vi "do all three.vi"(6 "Gyro Target":dbl, 7 "Max Time":dbl, 8 "X Target":dbl, 9 "Y Target":dbl, 10 "Encoders In":T1, 11 "PID Gains In":T2={"X PID"={"proportional gain (Kc)"=0.02000000000000001, "integral time (Ti, min)"=0.0, "derivative time (Td, min)"=0.0}, "Y PID"={"proportional gain (Kc)"=0.02000000000000001, "integral time (Ti, min)"=0.0, "derivative time (Td, min)"=0.0}, "Z PID"={"proportional gain (Kc)"=0.02000000000000001, "integral time (Ti, min)"=0.0, "derivative time (Td, min)"=0.0}} {"Z PID"."derivative time (Td, min)" format="%.3f"; "Z PID"."integral time (Ti, min)" format="%.3f"; "Z PID"."proportional gain (Kc)" format="%.3f"; "Y PID"."derivative time (Td, min)" format="%.3f"; "Y PID"."integral time (Ti, min)" format="%.3f"; "Y PID"."proportional gain (Kc)" format="%.3f"; "X PID"."derivative time (Td, min)" format="%.3f"; "X PID"."integral time (Ti, min)" format="%.3f"; "X PID"."proportional gain (Kc)" format="%.3f"}) -> (2 "Encoders Out":T1, 3 "PID Gains Out":T2={"X PID"={"proportional gain (Kc)"=0.02000000000000001, "integral time (Ti, min)"=0.0, "derivative time (Td, min)"=0.0}, "Y PID"={"proportional gain (Kc)"=0.02000000000000001, "integral time (Ti, min)"=0.0, "derivative time (Td, min)"=0.0}, "Z PID"={"proportional gain (Kc)"=0.02000000000000001, "integral time (Ti, min)"=0.0, "derivative time (Td, min)"=0.0}} {"Z PID"."derivative time (Td, min)" format="%.3f"; "Z PID"."integral time (Ti, min)" format="%.3f"; "Z PID"."proportional gain (Kc)" format="%.3f"; "Y PID"."derivative time (Td, min)" format="%.3f"; "Y PID"."integral time (Ti, min)" format="%.3f"; "Y PID"."proportional gain (Kc)" format="%.3f"; "X PID"."derivative time (Td, min)" format="%.3f"; "X PID"."integral time (Ti, min)" format="%.3f"; "X PID"."proportional gain (Kc)" format="%.3f"})   [LabVIEW 2018]
uses:
  <vilib>/addons/control/pid/NI_PID_pid.lvlib
  <vilib>/addons/control/pid/pid.llb/PID (DBL).vi
  Robot Global Data.vi
  SubSystems/Robot Information/Robot Information Global.vi
panel:
  in  "rest time":u32
  in  "Movement":enum16{"0", "1", "2", "3", "4", "5"}(ring)
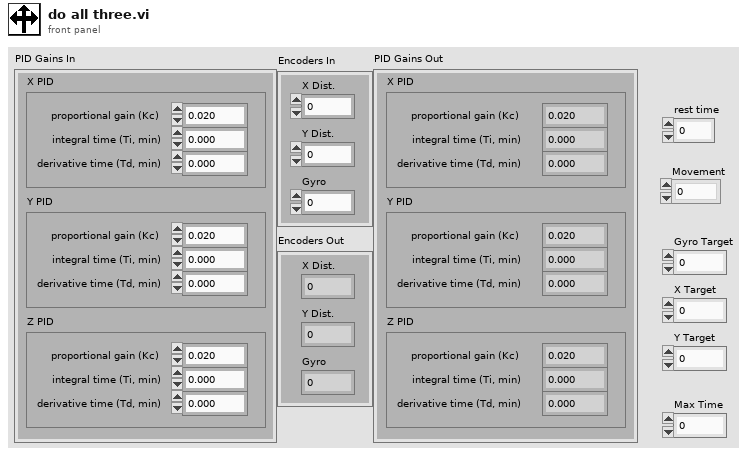
[diagram p1: front panel]
types:
  T1 = cluster{"X Dist.":dbl, "Y Dist.":dbl, "Gyro":dbl}
  T2 = cluster{"X PID":cluster{"proportional gain (Kc)":dbl, "integral time (Ti, min)":dbl, "derivative time (Td, min)":dbl}, "Y PID":cluster{"proportional gain (Kc)":dbl, "integral time (Ti, min)":dbl, "derivative time (Td, min)":dbl}, "Z PID":cluster{"proportional gain (Kc)":dbl, "integral time (Ti, min)":dbl, "derivative time (Td, min)":dbl}}
  T3 = enum16{"HP, Far-Top rocket, Lvl2 Right", "HP, Far-Top rocket, Lvl2 Left", "HP, Far-Top rocket, Lvl1 Right", "HP, Far-Top rocket, Lvl1 Left", "HP, Both-Top rocket, Lvl2 Right", "HP, Both-Top rocket, Lvl2 Left", "HP, Both-Top rocket, Lvl1 Right", "HP, Both-Top rocket, Lvl1 Left", "HP, Near cargo, Lvl2 ", "HP, Near cargo, Lvl1", "HP, Far cargo, Lvl2 ", "HP, Far cargo, Lvl1"}
  T4 = cluster{"proportional gain (Kc)":dbl, "integral time (Ti, min)":dbl, "derivative time (Td, min)":dbl}
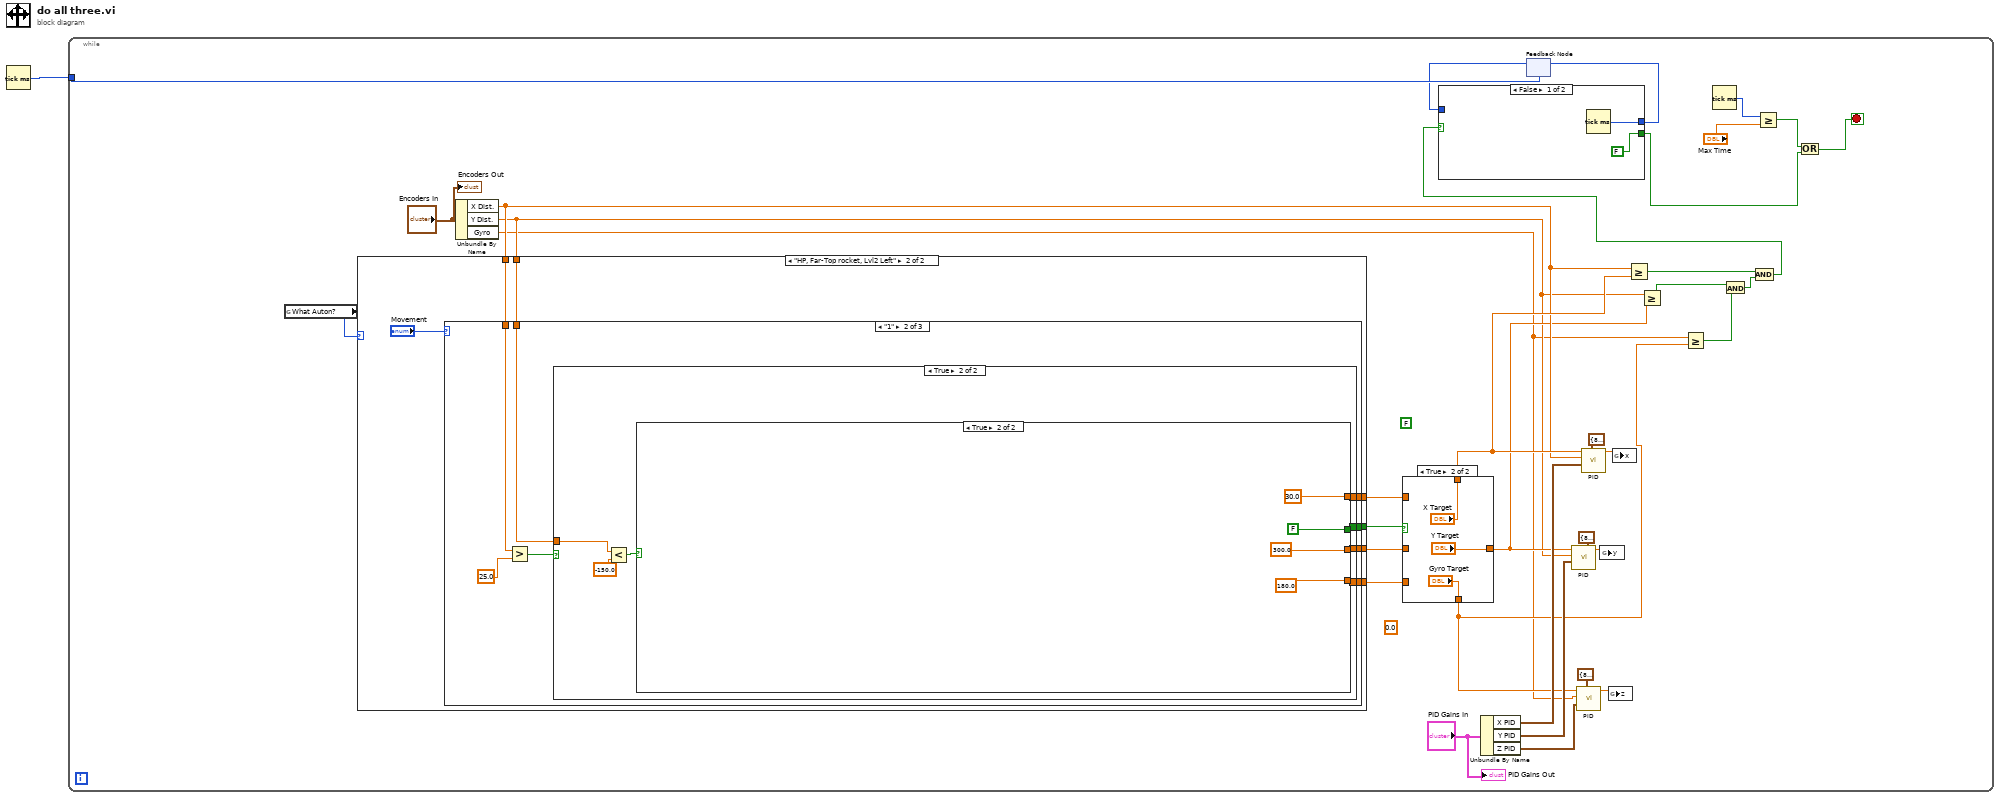
[diagram p0: block diagram]
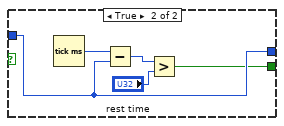
[diagram p2: hidden frame]
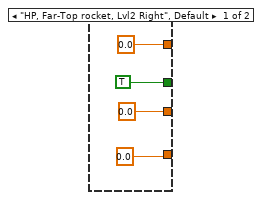
[diagram p4: hidden frame]
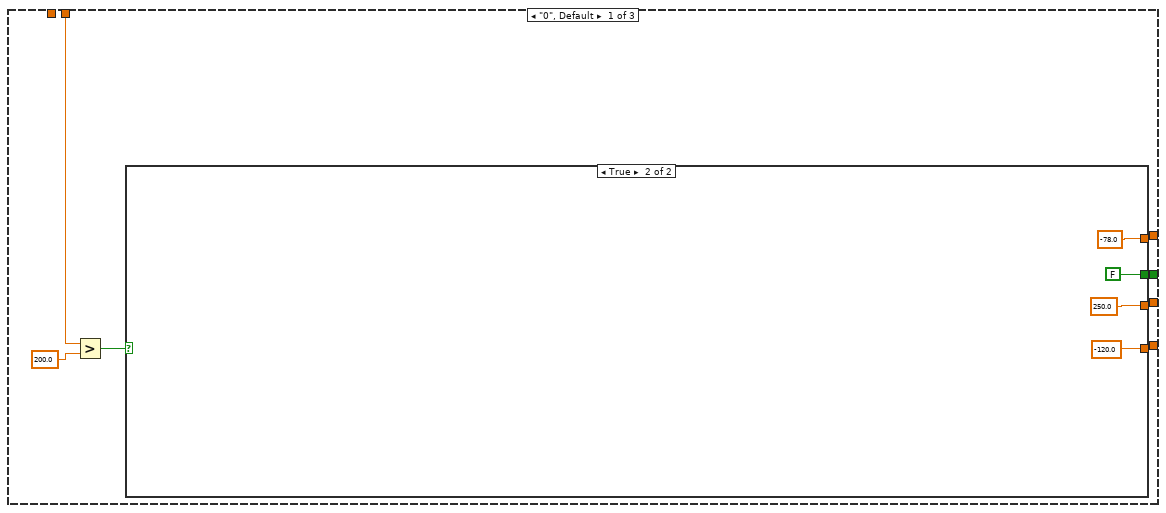
[diagram p5: hidden frame]
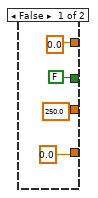
[diagram p6: hidden frame]
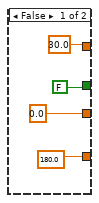
[diagram p7: hidden frame]
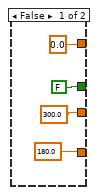
[diagram p8: hidden frame]
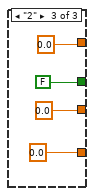
[diagram p9: hidden frame]
diagram:
  n1 = Tick Count (ms)() -> (millisecond timer value=w1:u32)
  n2 = while {
    tunnel: w1 -> [w5]
    stop <- w8 stop-if-true
    (unwired) 0.0
    (unwired) FALSE
    n3 = global read "Robot Information Global.vi" "What Auton?"() -> (w29:T3)
    n4 = Unbundle By Name("Encoders In") -> ("X Dist."=w17:dbl, "Y Dist."=w15:dbl, "Gyro"=w13:dbl)
    n5 = case shown="\"HP, Far-Top rocket, Lvl2 Left\"" w29 {
      tunnel: [0.0 w59] -> w22
      tunnel: [0.0 w58] -> w21
      tunnel: [0.0 w57] -> w20
      tunnel: w15 -> [_ w56]
      tunnel: [TRUE w55] -> w19
      tunnel: w17 -> [_ w54]
      frame "HP, Far-Top rocket, Lvl2 Right", Default {
      }
      frame "HP, Far-Top rocket, Lvl2 Left" {
        n6 = case shown="\"1\"" "Movement" {
          tunnel: [w66 w83 0.0] -> w59
          tunnel: [w65 w82 0.0] -> w58
          tunnel: [w64 w81 0.0] -> w57
          tunnel: w56 -> [w63 w76 _]
          tunnel: [w62 w80 FALSE] -> w55
          tunnel: w54 -> [_ w78 _]
          frame "0", Default {
            n7 = Greater?(x=w63, y=200.0) -> (0:w67:bool)
            n8 = case shown="True" w67 {
              tunnel: [0.0 -78.0] -> w66
              tunnel: [250.0 250.0] -> w65
              tunnel: [0.0 -120.0] -> w64
              tunnel: [FALSE FALSE] -> w62
              frame False {
              }
              frame True {
              }
            }
          }
          frame "1" {
            n9 = Greater?(x=w78, y=25.0) -> (0:w79:bool)
            n10 = case shown="True" w79 {
              tunnel: [30.0 w92] -> w83
              tunnel: [0.0 w94] -> w82
              tunnel: [180.0 w91] -> w81
              tunnel: [FALSE w93] -> w80
              tunnel: w76 -> [_ w89]
              frame False {
              }
              frame True {
                n11 = Less?(x=w89, y=-150.0) -> (x < y?=w90:bool)
                n12 = case shown="True" w90 {
                  tunnel: [300.0 300.0] -> w94
                  tunnel: [FALSE FALSE] -> w93
                  tunnel: [0.0 30.0] -> w92
                  tunnel: [180.0 180.0] -> w91
                  frame False {
                  }
                  frame True {
                  }
                }
              }
            }
          }
          frame "2" {
          }
        }
      }
    }
    n13 = case shown="True" w19 {
      tunnel: [w46 "X Target"] -> w18
      tunnel: [w45 "Y Target"] -> w16
      tunnel: [w44 "Gyro Target"] -> w14
      tunnel: w22 -> [w46 _]
      tunnel: w21 -> [w45 _]
      tunnel: w20 -> [w44 _]
      frame False {
      }
      frame True {
      }
    }
    n14 = Unbundle By Name("PID Gains In") -> ("X PID"=w27:T4, "Y PID"=w26:T4, "Z PID"=w25:T4)
    n15 = feedback #1(w5) -> (w4:u32)
    n16 = call-poly <vilib>:"PID.vi"("output range"=cluster{"output high":dbl, "output low":dbl} {"output high"=8.0, "output low"=-8.0}, "PID gains"=w26, "process variable"=w15, "setpoint"=w16) -> ("output"=w32:dbl)  [unwired: 6 in, 1 out]
    n17 = call-poly <vilib>:"PID.vi"("output range"=cluster{"output high":dbl, "output low":dbl} {"output high"=8.0, "output low"=-8.0}, "PID gains"=w25, "process variable"=w13, "setpoint"=w14) -> ("output"=w36:dbl)  [unwired: 6 in, 1 out]
    n18 = call-poly <vilib>:"PID.vi"("output range"=cluster{"output high":dbl, "output low":dbl} {"output high"=8.0, "output low"=-8.0}, "PID gains"=w27, "process variable"=w17, "setpoint"=w18) -> ("output"=w33:dbl)  [unwired: 6 in, 1 out]
    n19 = global write "Robot Global Data.vi" "y"(w32) -> ()
    n20 = global write "Robot Global Data.vi" "z"(w36) -> ()
    n21 = global write "Robot Global Data.vi" "x"(w33) -> ()
    n22 = Greater Or Equal?(x=w17, y=w18) -> (x >= y?=w12:bool)
    n23 = Greater Or Equal?(x=w15, y=w16) -> (x >= y?=w10:bool)
    n24 = Greater Or Equal?(x=w13, y=w14) -> (x >= y?=w9:bool)
    n25 = Tick Count (ms)() -> (millisecond timer value=w30:u32)
    n26 = And(x=w10, y=w9) -> (x .and. y?=w11:bool)
    n27 = And(x=w12, y=w11) -> (x .and. y?=w2:bool)
    n28 = case shown="False" w2 {
      tunnel: [w38 w41] -> w6
      tunnel: w4 -> [_ w41]
      tunnel: [FALSE w40] -> w3
      frame False {
        n29 = Tick Count (ms)() -> (millisecond timer value=w38:u32)
      }
      frame True {
        n30 = Tick Count (ms)() -> (millisecond timer value=w43:u32)
        n31 = Subtract(x=w43, y=w41) -> (x-y=w42:u32)
        n32 = Greater?(x=w42, y="rest time") -> (0:w40:bool)
      }
    }
    n33 = feedback-in #1(w6) -> ()
    n34 = Greater Or Equal?(x=w30, y="Max Time") -> (x >= y?=w7:bool)
    n35 = Or(x=w7, y=w3) -> (x .or. y?=w8:bool)
    "PID Gains Out" <- "PID Gains In"
    "Encoders Out" <- "Encoders In"
  }
